vi "Add Results Section.vi"(7 "MeasTable":refnum<vi>, 8 "error in":errorcluster, 11 "File refnum in":refnum<file>) -> (0 "error out":errorcluster, 3 "File refnum out":refnum<file>)   [LabVIEW 2021]
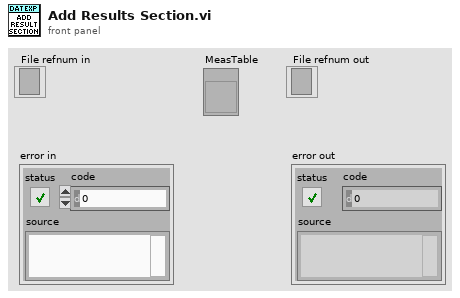
[diagram p1: front panel]
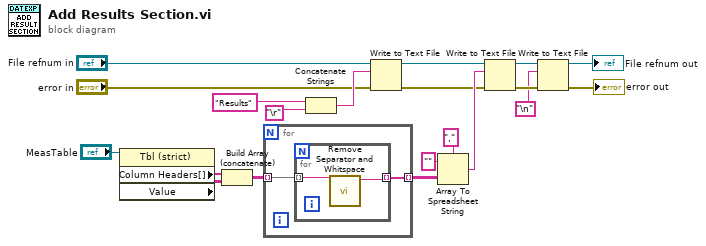
[diagram p0: block diagram]
diagram:
  n1 = property on="Property Node" class="Tbl (strict)"(reference="MeasTable") -> ("Column Headers[]"=w19:string[], "Value"=w18:string[][])  [unwired: 1 in, 2 out]
  n2 = Build Array (concatenate)(w19, w18) -> (w17:string[][])
  n3 = for {
    tunnel: w17 -> [w22] mode=indexing
    tunnel: [w21] -> w16 mode=indexing
    n4 = for {
      tunnel: w22 -> [w23] mode=indexing
      tunnel: [w24] -> w21 mode=indexing
      n5 = call "Remove Separator and Whitspace.vi"("Table string"=w23) -> ("Trimmed string"=w24:string)  [unwired: 10 in]
    }
  }
  n6 = Concatenate Strings("Results" ("element"), "\r") -> (w6:string)
  n7 = Write to Text File(file (use dialog)="File refnum in", text=w6, error in="error in") -> (refnum out=w20:refnum<file>, error out=w12:errorcluster)  [unwired: 1 in, 1 out]
  n8 = Array To Spreadsheet String(delimiter (Tab)=",", array=w16, 3:"" ("format string")) -> (spreadsheet string=w13:string)
  n9 = Write to Text File(file (use dialog)=w20, text=w13, error in=w12) -> (refnum out=w11:refnum<file>, error out=w10:errorcluster)  [unwired: 1 in, 1 out]
  n10 = Write to Text File(file (use dialog)=w11, text="\n", error in=w10) -> (refnum out=→"File refnum out":refnum<file>, error out=→"error out":errorcluster)  [unwired: 1 in, 1 out]
